vi "Read Camera Parameters.vi"(8 "error in (no error)":errorcluster, 11 "SOL Camera in":refnum<class "PL SOL Instruments Camera.lvclass">) -> (0 "error out":errorcluster, 2 "parameters":T1 {"prechanrge bus" items=["no", "yes"]; "Y read mode" items=["forward", "backward"]; "X read mode" items=["forward", "backward"]; "CCD advanced mode" items=["none", "nondestructive", "double slope"]; "CCD mode" items=["parallel", "serial", "low dark current", "large full well"]; "OUT2 mode" items=["exposure (negative)", "exposure (positive)", "delay before esposure (negative)", "delay after esposure (negative)", "external input inverted", "external input", "user register bit 1", "software start scan", "reserved"]; "OUT1 mode" items=["exposure (negative)", "exposure (positive)", "delay before esposure (negative)", "delay after esposure (negative)", "external input inverted", "external input", "user register bit 0", "software start scan", "reserved"]; "synchronization mode" items=["software"=0, "hardware"=1, "external rising edge type 1"=2, "external rising edge type 2"=3, "external falling edge type 1"=10, "external falling edge type 2"=11]; "bits per pixel" items=["8", "10", "12", "14", "16"]}, 3 "SOL Camera out":refnum<class "PL SOL Instruments Camera.lvclass">)   [LabVIEW 2015, in "PL SOL Instruments Camera.lvclass"]
doc: "Reads camera parameters."
uses:
  PL SOL Instruments Camera.lvclass
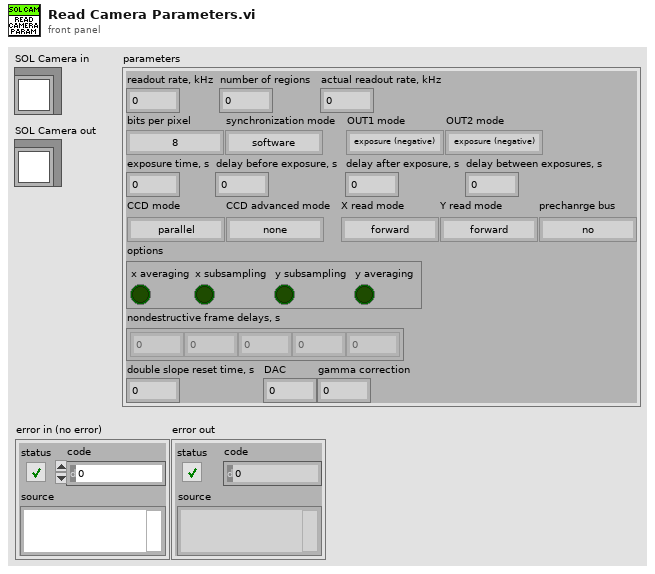
[diagram p1: front panel]
types:
  T1 = cluster{"number of regions":i32, "readout rate, kHz":i32, "actual readout rate, kHz":i32, "bits per pixel":u16, "synchronization mode":u16, "OUT1 mode":u16, "OUT2 mode":u16, "exposure time, s":dbl, "delay before exposure, s":dbl, "delay after exposure, s":dbl, "delay between exposures, s":dbl, "CCD mode":u16, "CCD advanced mode":u16, "X read mode":u16, "Y read mode":u16, "prechanrge bus":u16, "options":cluster{"x averaging":bool, "x subsampling":bool, "y subsampling":bool, "y averaging":bool}, "nondestructive frame delays, s":dbl[], "double slope reset time, s":dbl, "DAC":u16, "gamma correction":u16}
  T2 = cluster{"wCCDStandardMode":u16, "wCCDAdvancedMode":u16, "wXReadMode":u16, "wYReadMode":u16, "wPrechargeBus":u16, "wXOptions":u16}
  T3 = cluster{"wDSreset_Unit":u16, "wDSreset_Value":u16, "wDAC":u16, "wGammaCorrection":u16}
  T4 = cluster{"lRegNum":i32, "lReadoutSpeed":i32, "lFactReadoutSpeed":i32, "wBits":u16, "wSynchMode":u16, "wSynchOut1Type":u16, "wSynchOut2Type":u16}
  T5 = cluster{"wDSreset_Unit":u16, "wDSreset_Value":u16}
  T6 = cluster{"Boolean array[0]":bool, "Boolean array[1]":bool, "Boolean array[2]":bool, "Boolean array[3]":bool}
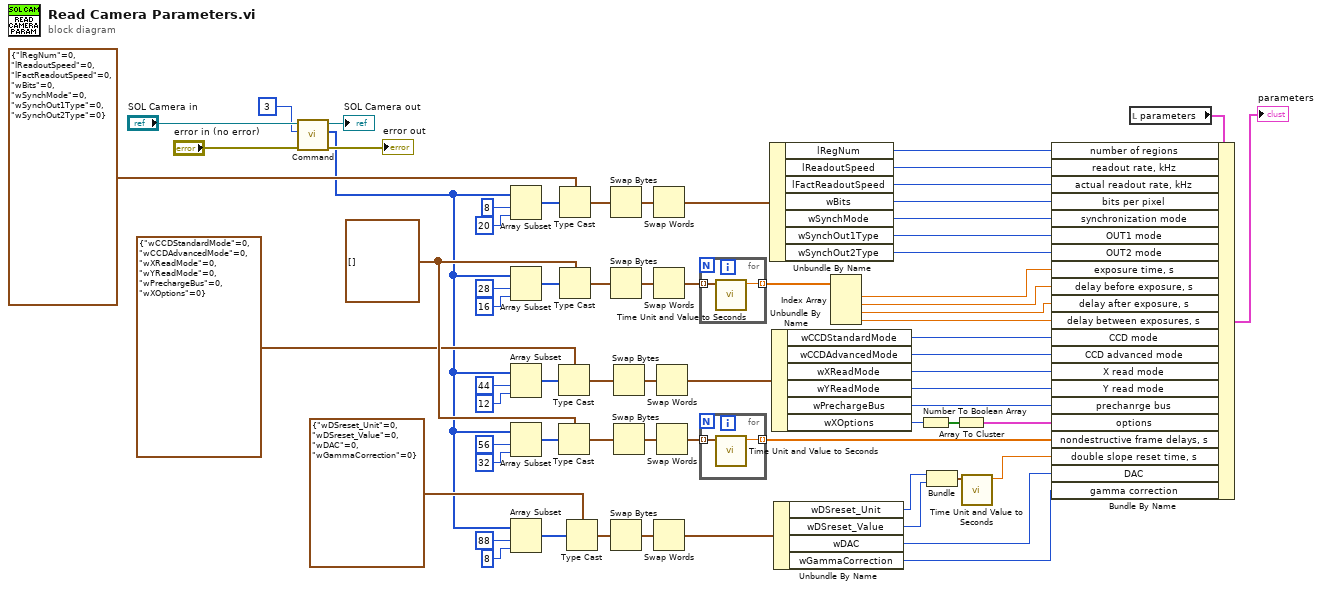
[diagram p0: block diagram]
diagram:
  w29 = cluster{"unit":u16, "value":u16}[] []
  n1 = call "Command.vi"("error in (no error)"="error in (no error)", "command"=u8 3, "SOL Camera in"="SOL Camera in") -> ("error out"=→"error out":errorcluster, "response"=w4:u8[], "SOL Camera out"=→"SOL Camera out":refnum<class "PL SOL Instruments Camera.lvclass">)  [unwired: 6 in]
  n2 = Array Subset(array=w4, index=8, length=20) -> (w63:u8[])
  n3 = Array Subset(array=w4, index=28, length=16) -> (w32:u8[])
  n4 = Array Subset(array=w4, index=44, length=12) -> (w57:u8[])
  n5 = Array Subset(array=w4, index=56, length=32) -> (w37:u8[])
  n6 = Array Subset(array=w4, index=88, length=8) -> (w52:u8[])
  n7 = Type Cast(type=T2 {"wCCDStandardMode"=0, "wCCDAdvancedMode"=0, "wXReadMode"=0, "wYReadMode"=0, "wPrechargeBus"=0, "wXOptions"=0} ("TPSICameraParamsV2 2"), x=w57) -> (*(type *) &x=w55:T2)
  n8 = Type Cast(type=w29, x=w37) -> (*(type *) &x=w39:cluster{"unit":u16, "value":u16}[])
  n9 = Type Cast(type=T4 {"lRegNum"=0, "lReadoutSpeed"=0, "lFactReadoutSpeed"=0, "wBits"=0, "wSynchMode"=0, "wSynchOut1Type"=0, "wSynchOut2Type"=0} ("TPSICameraParamsV2 2"), x=w63) -> (*(type *) &x=w60:T4)
  n10 = Type Cast(type=w29, x=w32) -> (*(type *) &x=w33:cluster{"unit":u16, "value":u16}[])
  n11 = Type Cast(type=T3 {"wDSreset_Unit"=0, "wDSreset_Value"=0, "wDAC"=0, "wGammaCorrection"=0}, x=w52) -> (*(type *) &x=w49:T3)
  n12 = Swap Bytes(anything=w60) -> (byte swapped=w59:T4)
  n13 = Swap Bytes(anything=w33) -> (byte swapped=w34:cluster{"unit":u16, "value":u16}[])
  n14 = Swap Bytes(anything=w49) -> (byte swapped=w50:T3)
  n15 = Swap Bytes(anything=w55) -> (byte swapped=w56:T2)
  n16 = Swap Bytes(anything=w39) -> (byte swapped=w38:cluster{"unit":u16, "value":u16}[])
  n17 = Swap Words(1:w59) -> (0:w58:T4)
  n18 = Swap Words(1:w34) -> (0:w27:cluster{"unit":u16, "value":u16}[])
  n19 = Swap Words(1:w50) -> (0:w12:T3)
  n20 = Swap Words(1:w56) -> (0:w23:T2)
  n21 = Swap Words(1:w38) -> (0:w14:cluster{"unit":u16, "value":u16}[])
  n22 = for {
    tunnel: w27 -> [w71] mode=indexing
    tunnel: [w70] -> w6 mode=indexing
    n23 = call "Time Unit and Value to Seconds.vi"("time unit and value"=w71) -> ("time, s"=w70:dbl)  [unwired: 10 in]
  }
  n24 = for {
    tunnel: w14 -> [w73] mode=indexing
    tunnel: [w72] -> w13 mode=indexing
    n25 = call "Time Unit and Value to Seconds.vi"("time unit and value"=w73) -> ("time, s"=w72:dbl)  [unwired: 10 in]
  }
  n26 = Unbundle By Name(w58) -> ("lRegNum"=w47:i32, "lReadoutSpeed"=w46:i32, "lFactReadoutSpeed"=w45:i32, "wBits"=w44:u16, "wSynchMode"=w43:u16, "wSynchOut1Type"=w42:u16, "wSynchOut2Type"=w41:u16)
  n27 = Unbundle By Name(w23) -> ("wCCDStandardMode"=w22:u16, "wCCDAdvancedMode"=w21:u16, "wXReadMode"=w20:u16, "wYReadMode"=w19:u16, "wPrechargeBus"=w18:u16, "wXOptions"=w17:u16)
  n28 = Unbundle By Name(w12) -> ("wDSreset_Unit"=w11:u16, "wDSreset_Value"=w10:u16, "wDAC"=w8:u16, "wGammaCorrection"=w9:u16)
  n29 = Index Array(array=w6) -> (element #1=w7:dbl, element #2=w26:dbl, element #3=w25:dbl, element #4=w24:dbl)  [unwired: 4 in]
  n30 = Number To Boolean Array(number=w17) -> (Boolean array=w16:bool[])
  n31 = Bundle("wDSreset_Unit"=w11, "wDSreset_Value"=w10) -> (w2:T5)  [unwired: 1 in]
  n32 = Array To Cluster(array=w16) -> (cluster=w15:T6)
  n33 = call "Time Unit and Value to Seconds.vi"("time unit and value"=w2) -> ("time, s"=w1:dbl)  [unwired: 10 in]
  n34 = local read "parameters"() -> (w48:T1)
  n35 = Bundle By Name(cluster=w48, "number of regions"=w47, "readout rate, kHz"=w46, "actual readout rate, kHz"=w45, "bits per pixel"=w44, "synchronization mode"=w43, "OUT1 mode"=w42, "OUT2 mode"=w41, "exposure time, s"=w7, "delay before exposure, s"=w26, "delay after exposure, s"=w25, "delay between exposures, s"=w24, "CCD mode"=w22, "CCD advanced mode"=w21, "X read mode"=w20, "Y read mode"=w19, "prechanrge bus"=w18, "options"=w15, "nondestructive frame delays, s"=w13, "double slope reset time, s"=w1, "DAC"=w8, "gamma correction"=w9) -> (→"parameters":T1)
